vi "Matlab Param Array to DBL.vi"(8 "error in (no error)":errorcluster, 10 "Name":string, 11 "Matlab Param Array":cluster{"Name":string, "Data":variant}[](array[cluster])) -> (0 "error out":errorcluster, 3 "data":dbl)   [LabVIEW 2014, in "Matlab API.lvlib"]
uses:
  Matlab API.lvlib
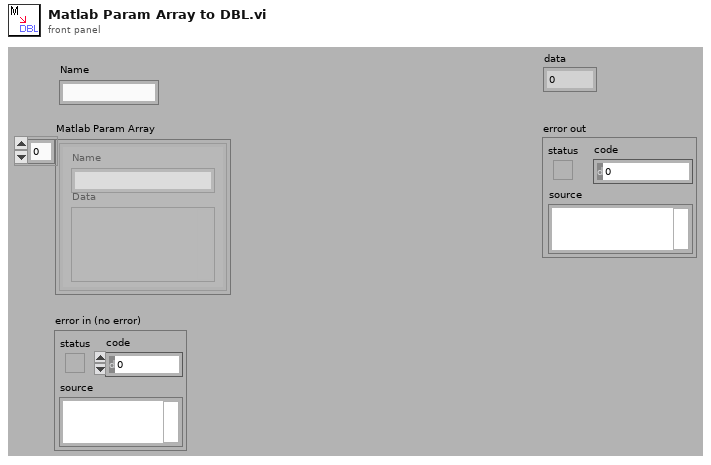
[diagram p1: front panel]
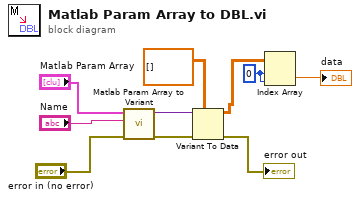
[diagram p0: block diagram]
diagram:
  w2 = 0 ("index (row)")
  n1 = call "Matlab Param Array to Variant.vi"("error in (no error)"="error in (no error)", "Name"="Name", "Variables"="Matlab Param Array") -> ("error out"=w9:errorcluster, "Data"=w10:variant)  [unwired: 7 out]
  n2 = Variant To Data(error in=w9, type=dbl[][] [], Variant=w10) -> (data=w3:dbl[][], error out=→"error out":errorcluster)
  n3 = Index Array(array=w3, index (row)=w2, index (col)=w2) -> (element=→"data":dbl)
